vi "Test Missing PPLs.vi"(11 "Test Case In":refnum<class "Missing in Project.lvclass">) -> (0 "error out":errorcluster, 3 "Test Case Out":refnum<class "Missing in Project.lvclass">)   [LabVIEW 2021, in "Missing in Project.lvclass"]
doc: "Tests to make sure all PPLs defined in the project are saved to disk."
uses:
  Missing in Project.lvclass
  C:/Program Files/National Instruments/LabVIEW 2024/vi.lib/Astemes/LUnit/Test Case.lvclass
  <vilib>/Astemes/LUnit/Test Case.lvclass/Test Case.ctl
  <vilib>/Astemes/LUnit/Core/LUnit Test Case/Private/Append Pass Result.vi
  <vilib>/Astemes/LUnit/Core/LUnit Test Case/Private/Append Fail Result.vi
  <vilib>/Astemes/LUnit/Core/LUnit Test Case/Private/Run In UI.vi
  <vilib>/Utility/error.llb/Clear Errors.vi
  <vilib>/Astemes/LUnit/Test Case.lvclass
panel:
  out "Missing items from LabVIEW project":path[](array[path])
  out "Pass":bool
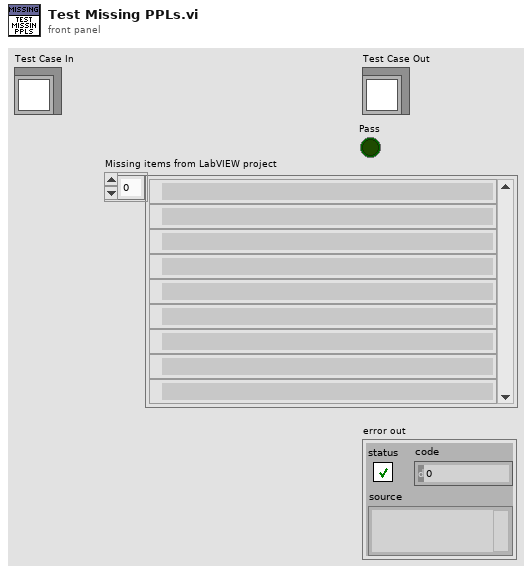
[diagram p1: front panel]
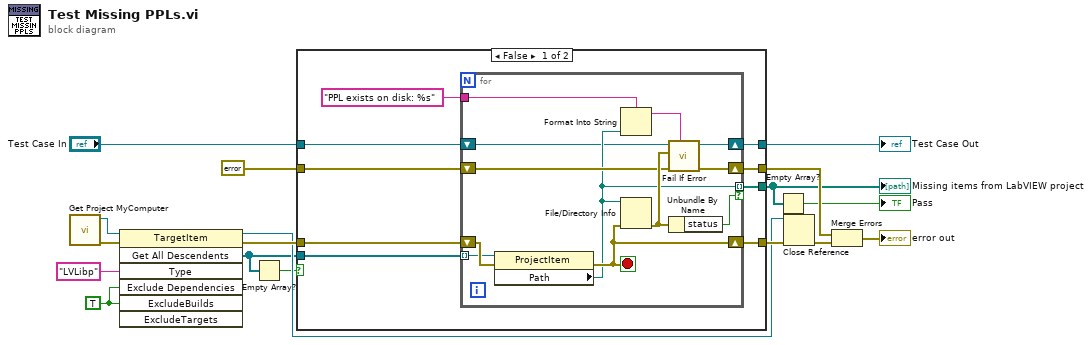
[diagram p0: block diagram]
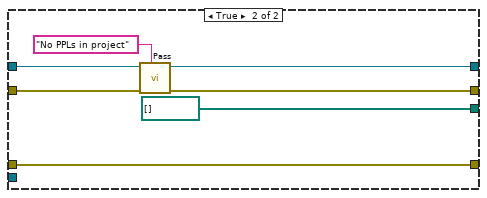
[diagram p2: hidden frame]
diagram:
  w1 = TRUE ("ExcludeBuilds")
  n1 = call "Get Project MyComputer.vi"() -> ("error out"=w13:errorcluster, "My Computer"=w6:refnum<vi>)  [unwired: 10 in]
  n2 = invoke class="TargetItem" method="Get All Descendents"(reference=w6, error in=w13, "Type"="LVLibp", "Exclude Dependencies"=w1, "ExcludeBuilds"=w1) -> (reference out=w9:refnum<vi>, error out=w17:errorcluster, "All Descendents"=w3:refnum<vi>[])  [unwired: 2 in, 4 out]
  n3 = Empty Array?(array=w3) -> (empty?=w2:bool)
  n4 = case shown="False" w2 {
    tunnel: w17 -> [w26 w43]
    tunnel: [w25 w43] -> w16
    tunnel: errorcluster {"status"=FALSE, "code"=0, "source"=""} ("error in (no error)") -> [w24 w44]
    tunnel: [w23 w45] -> w12
    tunnel: [w22 path[] []] -> w7
    tunnel: "Test Case In" -> [w20 w41]
    tunnel: [w19 w42] -> w4
    tunnel: w3 -> [w18 _]
    frame False {
      n5 = for {
        tunnel: w18 -> [w33] mode=indexing
        shift-right: [w36] -> w25
        shift-left: w26 -> [w37]
        tunnel: [w32] -> w22 mode=indexing if=w28
        shift-right: [w35] -> w23
        shift-left: w24 -> [w34]
        tunnel: "PPL exists on disk: %s" ("Label") -> [w31]
        shift-right: [w30] -> w19
        shift-left: w20 -> [w29]
        stop <- w36 stop-if-true
        n6 = property class="ProjectItem"(reference=w33, error in=w37) -> (error out=w36:errorcluster, "Path"=w32:path)  [unwired: 1 out]
        n7 = Format Into String(format string=w31, w32) -> (resulting string=w27:string)  [unwired: 2 in, 1 out]
        n8 = File/Directory Info(path=w32, error in=w36) -> (error out=w38:errorcluster)  [unwired: 6 out]
        n9 = call <vilib>:"Fail If Error.vi"("Description"=w27, "error in (no error)"=w34, "Assert error"=w38, "LUnit Test Case In"=w29) -> ("error out"=w35:errorcluster, "LUnit Test Case Out"=w30:refnum<class "Missing in Project.lvclass">)  [unwired: 6 in]
        n10 = Unbundle By Name(w38) -> ("status"=w28:bool)
      }
    }
    frame True {
      n11 = call <vilib>:"Pass.vi"("Description"="No PPLs in project", "error in (no error)"=w44, "LUnit Test Case In"=w41) -> ("error out"=w45:errorcluster, "LUnit Test Case Out"=w42:refnum<class "Missing in Project.lvclass">)  [unwired: 7 in]
    }
  }
  "Missing items from LabVIEW project" <- w7
  "Test Case Out" <- w4
  n12 = Empty Array?(array=w7) -> (empty?=→"Pass":bool)
  n13 = Close Reference(reference=w9, error in (no error)=w16) -> (error out=w15:errorcluster)
  n14 = Merge Errors(w12, w15) -> (→"error out":errorcluster)
